vi "менеджер отчетов.vi"(8 "String":string, 10 "data":string, 11 "path":path) -> ()   [LabVIEW 2016]
uses:
  <vilib>/Utility/file.llb/Read From Spreadsheet File (string).vi
  Granule-2000AT/PC/llb/Library.lvlib
panel:
  out "Waveform Graph":dbl[](graph)
  in  "диски":string(combo)
  out "PA1":string[](array[string])
  out "TP_gas":string[](array[string])
  out "TP roller":string[](array[string])
  out "TP 2.2":string[](array[string])
  out "TP 2.1":string[](array[string])
  out "TP 1.2":string[](array[string])
  out "TP_1.1":string[](array[string])
  out "PT3":string[](array[string])
  out "PT2":string[](array[string])
  out "PT1":string[](array[string])
  out "PE3":string[](array[string])
  out "PE2":string[](array[string])
  out "PE 1":string[](array[string])
  out "SP_speed_заг":string[](array[string])
  out "SP_speed_плазматрон":string[](array[string])
  out "V_заг":string[](array[string])
  out "U_ist":string[](array[string])
  out "I_ist":string[](array[string])
  out "PV":string[](array[string])
  out "data":string[](array[string])
  out "errors":string[][](array[string])
  out "all rows":string[][](array[string])
  in  "Изделия":string(combo)
  in  "Tab Control":T1(tab)
  out "PV зазор":cluster{"data dbl":dbl[], dbl[]}(graph)
  out "Speed":cluster{"data dbl":dbl[], dbl[]}[](graph)
  out "Rotation":cluster{"data dbl":dbl[], dbl[]}(graph)
  out "I_ист":cluster{"data dbl":dbl[], dbl[]}(graph)
  out "U_ист":cluster{"data dbl":dbl[], dbl[]}(graph)
  out "Vakuum":cluster{"data dbl":dbl[], dbl[]}[](graph)
  out "Temperature":cluster{"data dbl":dbl[], dbl[]}[](graph)
  out "Presure":cluster{"data dbl":dbl[], dbl[]}[](graph)
  out "Status":u8(slide) scale=0.0..4.0
  in  "Open Button":bool
  in  "Process Stop Button":bool
  in  "Blank Button":bool
  in  "Copy Button":bool
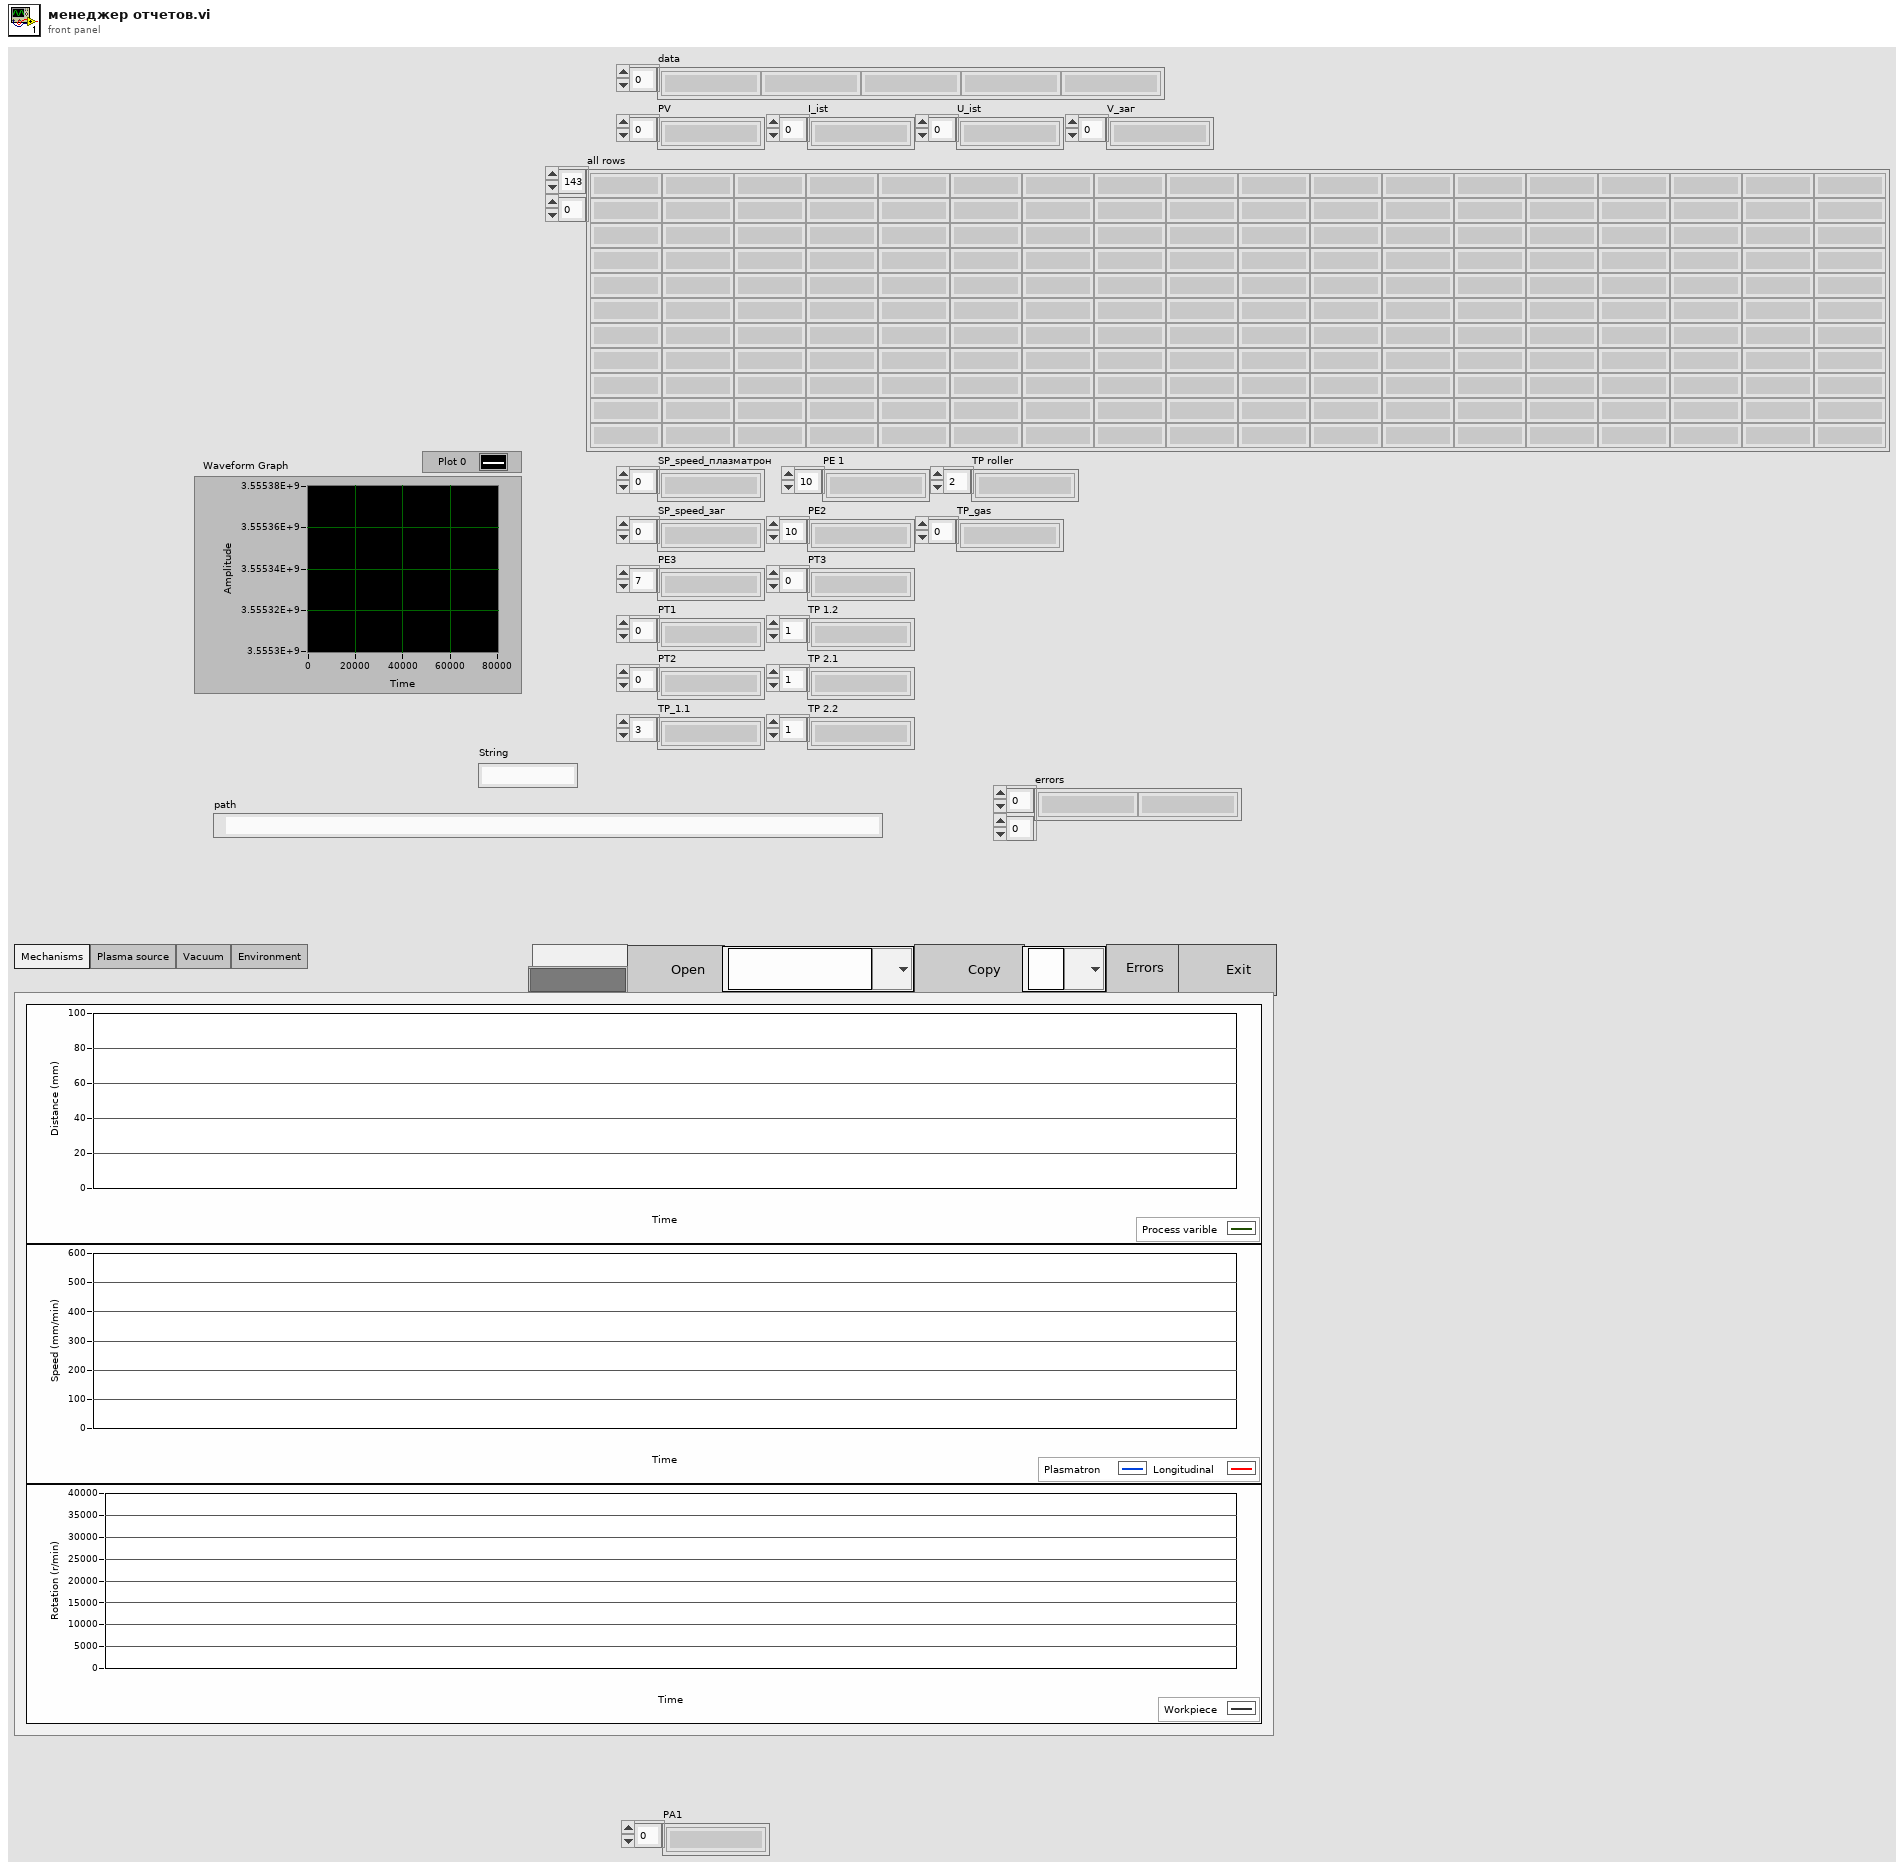
[diagram p1: front panel]
types:
  T1 = enum32{"Mechanisms", "Plasma source", "Vacuum", "Environment"}
  T2 = cluster{"String":string, "String":string, "String":string, cluster{"data dbl":dbl[], dbl[]}, cluster{"data dbl":dbl[], dbl[]}[], cluster{"data dbl":dbl[], dbl[]}}
  T3 = cluster{"String":string, "String":string, "String":string, cluster{"data dbl":dbl[], dbl[]}[], cluster{"data dbl":dbl[], dbl[]}[]}
  T4 = cluster{"String":string, "String":string, cluster{"data dbl":dbl[], dbl[]}, cluster{"data dbl":dbl[], dbl[]}, "String":string}
  T5 = cluster{"String":string, "String":string, "String":string, cluster{"data dbl":dbl[], dbl[]}[]}
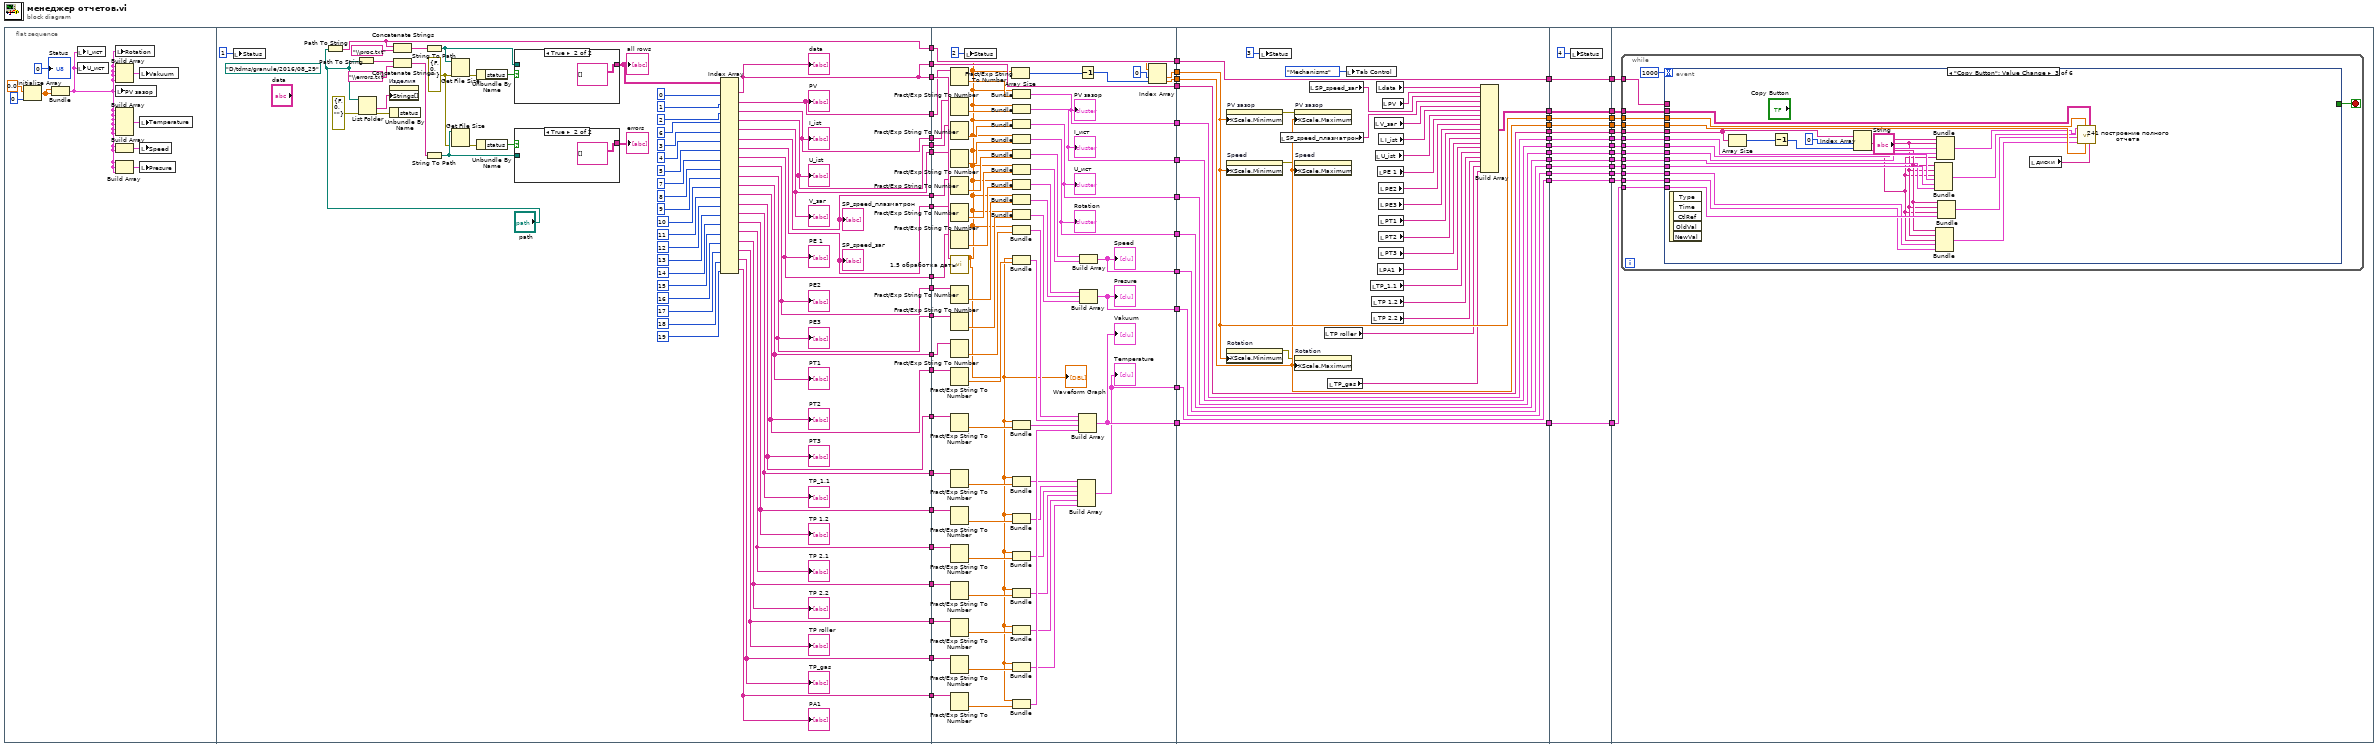
[diagram p0: block diagram]
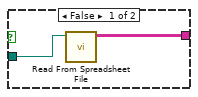
[diagram p2: hidden frame]
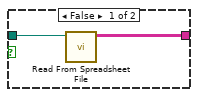
[diagram p3: hidden frame]
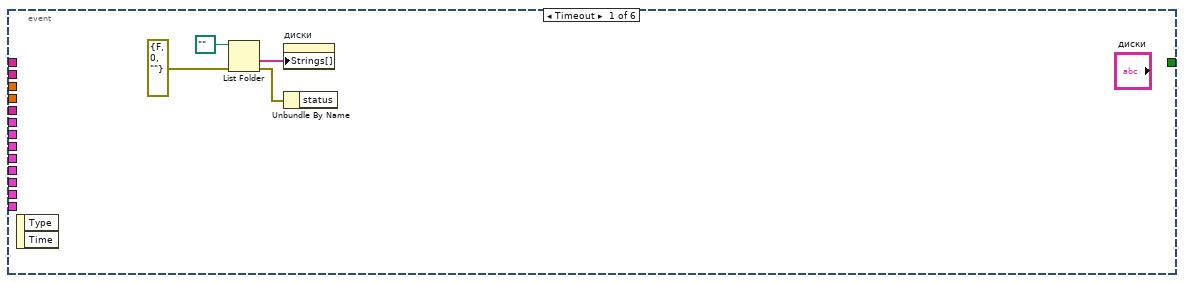
[diagram p4: hidden frame]
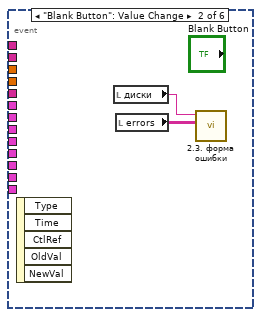
[diagram p5: hidden frame]
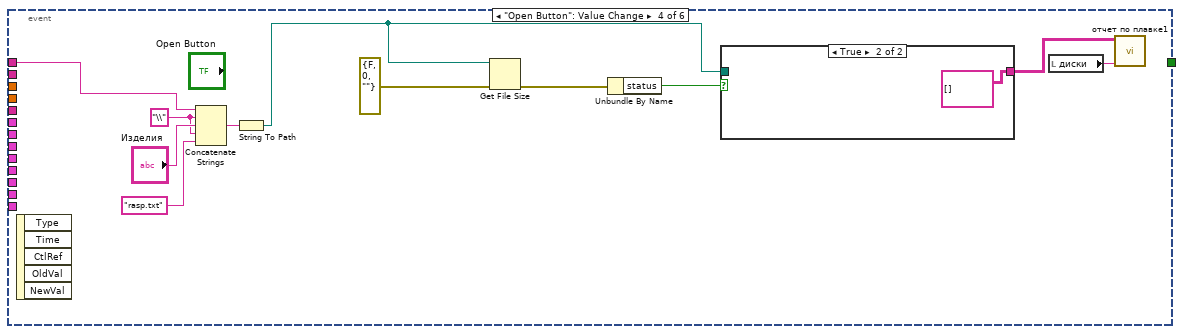
[diagram p6: hidden frame]
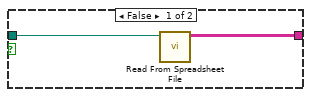
[diagram p7: hidden frame]
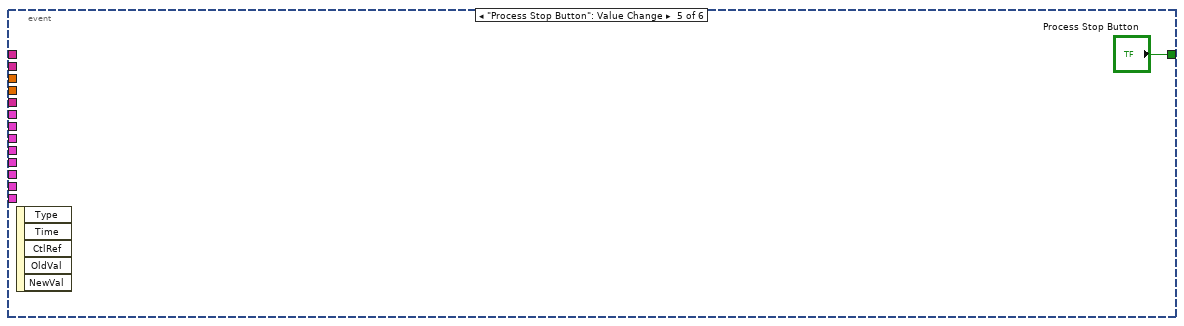
[diagram p8: hidden frame]
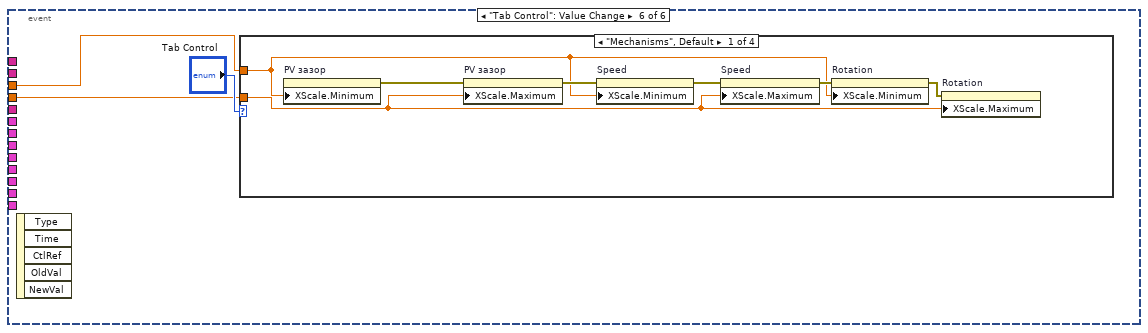
[diagram p9: hidden frame]
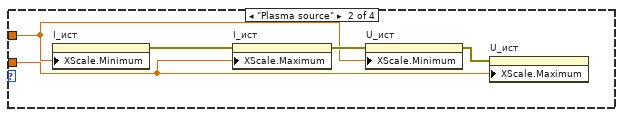
[diagram p10: hidden frame]
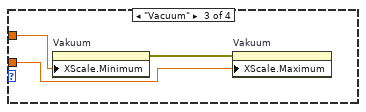
[diagram p11: hidden frame]
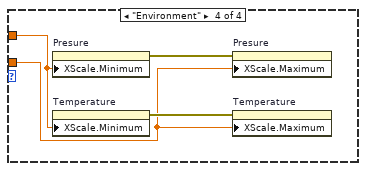
[diagram p12: hidden frame]
diagram:
  n1 = flat-sequence {
    tunnel: [w71] -> w60
    tunnel: [w93] -> w59
    tunnel: [w92] -> w58
    tunnel: [w91] -> w57
    tunnel: [w90] -> w56
    tunnel: [w89] -> w55
    tunnel: [w88] -> w54
    tunnel: [w87] -> w53
    tunnel: [w86] -> w52
    tunnel: [w85] -> w51
    tunnel: [w83] -> w50
    tunnel: [w82] -> w49
    tunnel: [w81] -> w48
    tunnel: [w80] -> w47
    tunnel: [w79] -> w46
    tunnel: [w78] -> w45
    tunnel: [w77] -> w44
    tunnel: [w76] -> w43
    tunnel: [w75] -> w42
    tunnel: [w74] -> w41
    tunnel: [w72] -> w37
    tunnel: [w71] -> w35
    tunnel: w60 -> [w206]
    tunnel: w59 -> [w205]
    tunnel: w58 -> [w200]
    tunnel: w57 -> [w198]
    tunnel: w56 -> [w194]
    tunnel: w55 -> [w192]
    tunnel: w54 -> [w189]
    tunnel: w53 -> [w188]
    tunnel: w52 -> [w186]
    tunnel: w51 -> [w184]
    tunnel: w50 -> [w175]
    tunnel: w49 -> [w174]
    tunnel: w48 -> [w173]
    tunnel: w47 -> [w172]
    tunnel: w46 -> [w155]
    tunnel: w45 -> [w154]
    tunnel: w44 -> [w153]
    tunnel: w43 -> [w152]
    tunnel: w42 -> [w151]
    tunnel: w41 -> [w150]
    tunnel: [w149] -> w40
    tunnel: [w148] -> w39
    tunnel: [w146] -> w38
    tunnel: w37 -> [w146]
    tunnel: [w145] -> w36
    tunnel: w35 -> [w145]
    tunnel: [w144] -> w22
    tunnel: [w143] -> w19
    tunnel: [w142] -> w16
    tunnel: [w141] -> w13
    tunnel: [w140] -> w10
    tunnel: [w139] -> w7
    tunnel: [w138] -> w4
    tunnel: [w137] -> w1
    tunnel: w40 -> [w242]
    tunnel: [w242] -> w34
    tunnel: w39 -> [w241]
    tunnel: [w241] -> w32
    tunnel: [w236] -> w30
    tunnel: w38 -> [w236]
    tunnel: [w216] -> w28
    tunnel: [w215] -> w26
    tunnel: w36 -> [w215]
    tunnel: [w214] -> w23
    tunnel: w22 -> [w214]
    tunnel: [w213] -> w20
    tunnel: w19 -> [w213]
    tunnel: [w212] -> w17
    tunnel: w16 -> [w212]
    tunnel: [w211] -> w14
    tunnel: w13 -> [w211]
    tunnel: [w210] -> w11
    tunnel: w10 -> [w210]
    tunnel: [w209] -> w8
    tunnel: w7 -> [w209]
    tunnel: [w208] -> w5
    tunnel: w4 -> [w208]
    tunnel: [w207] -> w2
    tunnel: w1 -> [w207]
    tunnel: w34 -> [w257]
    tunnel: [w257] -> w33
    tunnel: w32 -> [w256]
    tunnel: [w256] -> w31
    tunnel: w30 -> [w255]
    tunnel: [w255] -> w29
    tunnel: w28 -> [w254]
    tunnel: [w254] -> w27
    tunnel: w26 -> [w253]
    tunnel: [w253] -> w25
    tunnel: [w251] -> w24
    tunnel: w23 -> [w251]
    tunnel: [w250] -> w21
    tunnel: w20 -> [w250]
    tunnel: [w249] -> w18
    tunnel: w17 -> [w249]
    tunnel: [w248] -> w15
    tunnel: w14 -> [w248]
    tunnel: [w247] -> w12
    tunnel: w11 -> [w247]
    tunnel: [w246] -> w9
    tunnel: w8 -> [w246]
    tunnel: [w245] -> w6
    tunnel: w5 -> [w245]
    tunnel: [w244] -> w3
    tunnel: w2 -> [w244]
    tunnel: w33 -> [w270]
    tunnel: w31 -> [w269]
    tunnel: w29 -> [w268]
    tunnel: w27 -> [w267]
    tunnel: w25 -> [w266]
    tunnel: w24 -> [w265]
    tunnel: w21 -> [w264]
    tunnel: w18 -> [w263]
    tunnel: w15 -> [w262]
    tunnel: w12 -> [w261]
    tunnel: w9 -> [w260]
    tunnel: w6 -> [w259]
    tunnel: w3 -> [w258]
    frame #0 {
      n2 = Initialize Array(0.0, 0 ("dimension size")) -> (w67:dbl[])
      n3 = Bundle(w67, w67) -> (w63:cluster{dbl[], dbl[]})  [unwired: 1 in]
      n4 = local write "I_ист"(w63) -> ()
      n5 = local write "U_ист"(w63) -> ()
      n6 = local write "Rotation"(w63) -> ()
      n7 = Build Array(w63, w63, w63, w63) -> (w64:cluster{dbl[], dbl[]}[])
      n8 = local write "PV зазор"(w63) -> ()
      n9 = Build Array(w63, w63, w63, w63, w63, w63) -> (w62:cluster{dbl[], dbl[]}[])
      n10 = Build Array(w63, w63) -> (w66:cluster{dbl[], dbl[]}[])
      n11 = Build Array(w63, w63, w63) -> (w65:cluster{dbl[], dbl[]}[])
      n12 = local write "Vakuum"(w64) -> ()
      n13 = local write "Temperature"(w62) -> ()
      n14 = local write "Speed"(w66) -> ()
      n15 = local write "Presure"(w65) -> ()
      "Status" <- u8 0 ("Status")
    }
    frame #1 {
      w114 = errorcluster {"status"=FALSE, "code"=0, "source"=""} ("error in")
      (unwired) path "D:/tdms/granule/2016/08_29" ("path")
      n16 = local write "Status"(u8 1 ("Status")) -> ()
      n17 = Path To String(path="path") -> (string=w72:string)
      n18 = Path To String(path="path") -> (string=w125:string)
      n19 = List Folder(path="path", error in=errorcluster {"status"=FALSE, "code"=0, "source"=""}) -> (folder names=w127:string[], error out=w128:errorcluster)  [unwired: 2 in, 2 out]
      n20 = property on="Изделия" class="CmbBox"("Strings[]"=w127) -> ()  [unwired: 2 in, 2 out]
      n21 = Unbundle By Name(w128) -> ()  [unwired: 1 out]
      n22 = Concatenate Strings(w72, "\\proc.txt" ("string")) -> (w123:string)
      n23 = Concatenate Strings(w125, "\\errors.txt" ("string")) -> (w122:string)
      n24 = String To Path(string=w123) -> (path=w121:path)
      n25 = String To Path(string=w122) -> (path=w115:path)
      n26 = Get File Size(file=w121, error in=w114) -> (0:w120:errorcluster)  [unwired: 2 out]
      n27 = Get File Size(file=w115, error in=w114) -> (0:w117:errorcluster)  [unwired: 2 out]
      n28 = Unbundle By Name(w120) -> ("status"=w119:bool)
      n29 = Unbundle By Name(w117) -> ("status"=w116:bool)
      n30 = case shown="True" w119 {
        tunnel: w121 -> [w134 _]
        tunnel: [w133 string[][] [] ("all rows")] -> w113
        frame False {
          n31 = call-poly <vilib>:"Read From Spreadsheet File.vi"("file path (dialog if empty)"=w134) -> ("all rows"=w133:string[][])  [unwired: 6 in, 4 out]
        }
        frame True {
        }
      }
      "all rows" <- w113
      n32 = case shown="True" w116 {
        tunnel: w115 -> [w131 _]
        tunnel: [w130 string[][] [] ("all rows")] -> w118
        frame False {
          n33 = call-poly <vilib>:"Read From Spreadsheet File.vi"("file path (dialog if empty)"=w131) -> ("all rows"=w130:string[][])  [unwired: 6 in, 4 out]
        }
        frame True {
        }
      }
      "errors" <- w118
      n34 = Index Array(array=w113, index (col) #1=0 ("disabled index (col)"), index (col) #2=1 ("index (col)"), index (col) #3=2 ("index (col)"), index (col) #4=6 ("index (col)"), index (col) #5=3 ("index (col)"), index (col) #6=4 ("index (col)"), index (col) #7=5 ("index (col)"), index (col) #8=7 ("index (col)"), index (col) #9=8 ("index (col)"), index (col) #10=9 ("index (col)"), index (col) #11=10 ("index (col)"), index (col) #12=11 ("index (col)"), index (col) #13=12 ("index (col)"), index (col) #14=13 ("index (col)"), index (col) #15=14 ("index (col)"), index (col) #16=15 ("index (col)"), index (col) #17=16 ("index (col)"), index (col) #18=17 ("index (col)"), index (col) #19=18 ("index (col)"), index (col) #20=19 ("index (col)")) -> (element #1=w71:string[], element #2=w93:string[], element #3=w89:string[], element #4=w88:string[], element #5=w90:string[], element #6=w92:string[], element #7=w91:string[], element #8=w87:string[], element #9=w86:string[], element #10=w85:string[], element #11=w80:string[], element #12=w81:string[], element #13=w82:string[], element #14=w79:string[], element #15=w78:string[], element #16=w77:string[], element #17=w76:string[], element #18=w75:string[], element #19=w74:string[], element #20=w83:string[])  [unwired: 20 in]
      "data" <- w71
      "PV" <- w93
      "I_ist" <- w89
      "U_ist" <- w88
      "V_заг" <- w90
      "SP_speed_плазматрон" <- w92
      "SP_speed_заг" <- w91
      "PE 1" <- w87
      "PE2" <- w86
      "PE3" <- w85
      "PT1" <- w80
      "PT2" <- w81
      "PT3" <- w82
      "TP_1.1" <- w79
      "TP 1.2" <- w78
      "TP 2.1" <- w77
      "TP 2.2" <- w76
      "TP roller" <- w75
      "TP_gas" <- w74
      "PA1" <- w83
    }
    frame #2 {
      n35 = Fract/Exp String To Number(string=w205) -> (number=w201:dbl[])  [unwired: 3 in, 1 out]
      n36 = Fract/Exp String To Number(string=w192) -> (number=w191:dbl[])  [unwired: 3 in, 1 out]
      n37 = Fract/Exp String To Number(string=w189) -> (number=w190:dbl[])  [unwired: 3 in, 1 out]
      n38 = Fract/Exp String To Number(string=w194) -> (number=w193:dbl[])  [unwired: 3 in, 1 out]
      n39 = Fract/Exp String To Number(string=w200) -> (number=w199:dbl[])  [unwired: 3 in, 1 out]
      n40 = Fract/Exp String To Number(string=w198) -> (number=w197:dbl[])  [unwired: 3 in, 1 out]
      n41 = Fract/Exp String To Number(string=w188) -> (number=w187:dbl[])  [unwired: 3 in, 1 out]
      n42 = call "1.5 обработка даты.vi"("data"=w206) -> ("data dbl"=w136:dbl[])  [unwired: 10 in]
      "Waveform Graph" <- w136
      n43 = Fract/Exp String To Number(string=w186) -> (number=w185:dbl[])  [unwired: 3 in, 1 out]
      n44 = Fract/Exp String To Number(string=w184) -> (number=w183:dbl[])  [unwired: 3 in, 1 out]
      n45 = Fract/Exp String To Number(string=w172) -> (number=w168:dbl[])  [unwired: 3 in, 1 out]
      n46 = Fract/Exp String To Number(string=w173) -> (number=w169:dbl[])  [unwired: 3 in, 1 out]
      n47 = Fract/Exp String To Number(string=w174) -> (number=w170:dbl[])  [unwired: 3 in, 1 out]
      n48 = Fract/Exp String To Number(string=w155) -> (number=w161:dbl[])  [unwired: 3 in, 1 out]
      n49 = Fract/Exp String To Number(string=w154) -> (number=w160:dbl[])  [unwired: 3 in, 1 out]
      n50 = Fract/Exp String To Number(string=w153) -> (number=w159:dbl[])  [unwired: 3 in, 1 out]
      n51 = Fract/Exp String To Number(string=w152) -> (number=w158:dbl[])  [unwired: 3 in, 1 out]
      n52 = Fract/Exp String To Number(string=w151) -> (number=w156:dbl[])  [unwired: 3 in, 1 out]
      n53 = Fract/Exp String To Number(string=w150) -> (number=w157:dbl[])  [unwired: 3 in, 1 out]
      n54 = Fract/Exp String To Number(string=w175) -> (number=w171:dbl[])  [unwired: 3 in, 1 out]
      n55 = local write "Status"(u8 2 ("Status")) -> ()
      n56 = Array Size(array=w136) -> (size(s)=w203:i32)
      n57 = Bundle("data dbl"=w136, w201) -> (w144:cluster{"data dbl":dbl[], dbl[]})  [unwired: 1 in]
      "PV зазор" <- w144
      n58 = Bundle("data dbl"=w136, w191) -> (w141:cluster{"data dbl":dbl[], dbl[]})  [unwired: 1 in]
      "I_ист" <- w141
      n59 = Bundle("data dbl"=w136, w190) -> (w140:cluster{"data dbl":dbl[], dbl[]})  [unwired: 1 in]
      "U_ист" <- w140
      n60 = Bundle("data dbl"=w136, w193) -> (w142:cluster{"data dbl":dbl[], dbl[]})  [unwired: 1 in]
      "Rotation" <- w142
      n61 = Bundle("data dbl"=w136, w199) -> (w196:cluster{"data dbl":dbl[], dbl[]})  [unwired: 1 in]
      n62 = Bundle("data dbl"=w136, w197) -> (w195:cluster{"data dbl":dbl[], dbl[]})  [unwired: 1 in]
      n63 = Bundle("data dbl"=w136, w187) -> (w182:cluster{"data dbl":dbl[], dbl[]})  [unwired: 1 in]
      n64 = Bundle("data dbl"=w136, w185) -> (w181:cluster{"data dbl":dbl[], dbl[]})  [unwired: 1 in]
      n65 = Bundle("data dbl"=w136, w183) -> (w180:cluster{"data dbl":dbl[], dbl[]})  [unwired: 1 in]
      n66 = Bundle("data dbl"=w136, w168) -> (w179:cluster{"data dbl":dbl[], dbl[]})  [unwired: 1 in]
      n67 = Bundle("data dbl"=w136, w169) -> (w178:cluster{"data dbl":dbl[], dbl[]})  [unwired: 1 in]
      n68 = Bundle("data dbl"=w136, w170) -> (w177:cluster{"data dbl":dbl[], dbl[]})  [unwired: 1 in]
      n69 = Bundle("data dbl"=w136, w161) -> (w167:cluster{"data dbl":dbl[], dbl[]})  [unwired: 1 in]
      n70 = Bundle("data dbl"=w136, w160) -> (w166:cluster{"data dbl":dbl[], dbl[]})  [unwired: 1 in]
      n71 = Bundle("data dbl"=w136, w159) -> (w165:cluster{"data dbl":dbl[], dbl[]})  [unwired: 1 in]
      n72 = Bundle("data dbl"=w136, w158) -> (w164:cluster{"data dbl":dbl[], dbl[]})  [unwired: 1 in]
      n73 = Bundle("data dbl"=w136, w156) -> (w163:cluster{"data dbl":dbl[], dbl[]})  [unwired: 1 in]
      n74 = Bundle("data dbl"=w136, w157) -> (w162:cluster{"data dbl":dbl[], dbl[]})  [unwired: 1 in]
      n75 = Bundle("data dbl"=w136, w171) -> (w176:cluster{"data dbl":dbl[], dbl[]})  [unwired: 1 in]
      n76 = Build Array(w167, w166, w165, w164, w163, w162) -> (w137:cluster{"data dbl":dbl[], dbl[]}[])
      "Temperature" <- w137
      n77 = Decrement(x=w203) -> (x-1=w202:i32)
      n78 = Build Array(w179, w178, w177, w176) -> (w139:cluster{"data dbl":dbl[], dbl[]}[])
      "Vakuum" <- w139
      n79 = Build Array(w182, w181, w180) -> (w138:cluster{"data dbl":dbl[], dbl[]}[])
      "Presure" <- w138
      n80 = Build Array(w196, w195) -> (w143:cluster{"data dbl":dbl[], dbl[]}[])
      "Speed" <- w143
      n81 = Index Array(array=w136, index #1=0 ("index"), index #2=w202) -> (element #1=w149:dbl, element #2=w148:dbl)
    }
    frame #3 {
      n82 = property on="PV зазор" class="XYGraph (strict)"("XScale.Minimum"=w242) -> (error out=w240:errorcluster)  [unwired: 2 in, 1 out]
      n83 = property on="Speed" class="XYGraph (strict)"("XScale.Minimum"=w242) -> (error out=w239:errorcluster)  [unwired: 2 in, 1 out]
      n84 = property on="Rotation" class="XYGraph (strict)"("XScale.Minimum"=w242) -> (error out=w238:errorcluster)  [unwired: 2 in, 1 out]
      n85 = local write "Status"(u8 3 ("Status")) -> ()
      n86 = local read "SP_speed_плазматрон"() -> (w232:string[])
      n87 = property on="PV зазор" class="XYGraph (strict)"(error in=w240, "XScale.Maximum"=w241) -> ()  [unwired: 1 in, 2 out]
      n88 = property on="Speed" class="XYGraph (strict)"(error in=w239, "XScale.Maximum"=w241) -> ()  [unwired: 1 in, 2 out]
      n89 = property on="Rotation" class="XYGraph (strict)"(error in=w238, "XScale.Maximum"=w241) -> ()  [unwired: 1 in, 2 out]
      n90 = local read "SP_speed_заг"() -> (w233:string[])
      n91 = local read "TP roller"() -> (w218:string[])
      n92 = local read "TP_gas"() -> (w217:string[])
      n93 = local write "Tab Control"(T1."Mechanisms" ("Tab Control")) -> ()
      n94 = local read "TP_1.1"() -> (w221:string[])
      n95 = local read "TP 1.2"() -> (w220:string[])
      n96 = local read "TP 2.2"() -> (w219:string[])
      n97 = local read "V_заг"() -> (w231:string[])
      n98 = local read "U_ist"() -> (w229:string[])
      n99 = local read "data"() -> (w235:string[])
      n100 = local read "PE 1"() -> (w228:string[])
      n101 = local read "PA1"() -> (w222:string[])
      n102 = local read "I_ist"() -> (w230:string[])
      n103 = local read "PE2"() -> (w227:string[])
      n104 = local read "PE3"() -> (w226:string[])
      n105 = local read "PT1"() -> (w225:string[])
      n106 = local read "PT2"() -> (w224:string[])
      n107 = local read "PT3"() -> (w223:string[])
      n108 = local read "PV"() -> (w234:string[])
      n109 = Build Array(w235, w234, w233, w232, w231, w230, w229, w228, w227, w226, w225, w224, w223, w222, w221, w220, w219, w218, w217) -> (w216:string[][])
    }
    frame #4 {
      n110 = local write "Status"(u8 4 ("Status")) -> ()
    }
    frame #5 {
      n111 = while {
        tunnel: w270 -> [w285]
        tunnel: w269 -> [w284]
        tunnel: w268 -> [w282]
        tunnel: w267 -> [w280]
        tunnel: w266 -> [w279]
        tunnel: w265 -> [w278]
        tunnel: w264 -> [w277]
        tunnel: w263 -> [w276]
        tunnel: w262 -> [w275]
        tunnel: w261 -> [w274]
        tunnel: w260 -> [w273]
        tunnel: w259 -> [w272]
        tunnel: w258 -> [w271]
        stop <- w281 stop-if-true
        n112 = event shown="[2] \"Copy Button\": Value Change" {
          selector: _ -> [_ _ _ _ _ _]
          dyn-events: _ -> [_ _ _ _ _ _]
          timeout: 1000 -> [_ _ _ _ _ _]
          tunnel: w285 -> [_ _ w312 _ _ w331]
          tunnel: w284 -> [_ _ w313 _ _ w330]
          tunnel: w282 -> [_ _ _ w325 _ _]
          tunnel: [_ _ _ _ "Process Stop Button" _] -> w281
          tunnel: w280 -> [_ _ w314 _ _ _]
          tunnel: w279 -> [_ _ w310 _ _ _]
          tunnel: w278 -> [_ _ w306 _ _ _]
          tunnel: w277 -> [_ _ w305 _ _ _]
          tunnel: w276 -> [_ _ w304 _ _ _]
          tunnel: w275 -> [_ _ w302 _ _ _]
          tunnel: w274 -> [_ _ w301 _ _ _]
          tunnel: w273 -> [_ _ w299 _ _ _]
          tunnel: w272 -> [_ _ w295 _ _ _]
          tunnel: w271 -> [_ _ w294 _ _ _]
          event Timeout {
            n113 = event-data() -> ()  [unwired: 1 in, 2 out]
            n114 = List Folder(path=path "", error in=errorcluster {"status"=FALSE, "code"=0, "source"=""}) -> (folder names=w288:string[], error out=w286:errorcluster)  [unwired: 2 in, 2 out]
            n115 = property on="диски" class="CmbBox"("Strings[]"=w288) -> ()  [unwired: 2 in, 2 out]
            n116 = Unbundle By Name(w286) -> ()  [unwired: 1 out]
          }
          event "Blank Button": Value Change {
            n117 = event-data() -> ()  [unwired: 1 in, 5 out]
            n118 = local read "диски"() -> (w291:string)
            n119 = local read "errors"() -> (w290:string[][])
            n120 = call "2.3. форма ошибки.vi"("errors"=w290, "disk"=w291) -> ()  [unwired: 10 in]
          }
          event "Copy Button": Value Change {
            n121 = event-data() -> ()  [unwired: 1 in, 5 out]
            n122 = Array Size(array=w310) -> (size(s)=w308:i32)
            n123 = Decrement(x=w308) -> (x-1=w307:i32)
            n124 = Index Array(array=w310, index #1=0 ("index"), index #2=w307) -> (element #1=w296:string, element #2=w297:string)
            n125 = Bundle("String"=w297, "String"=w296, "String"="String", w306, w305, w304) -> (w303:T2)  [unwired: 1 in]
            n126 = Bundle("String"=w297, "String"=w296, "String"="String", w295, w294) -> (w293:T3)  [unwired: 1 in]
            n127 = Bundle("String"=w297, "String"=w296, w302, w301, "String"="String") -> (w300:T4)  [unwired: 1 in]
            n128 = Bundle("String"=w297, "String"=w296, "String"="String", w299) -> (w298:T5)  [unwired: 1 in]
            n129 = local read "диски"() -> (w311:string)
            n130 = call "241 построение полного отчета.vi"("disk"=w311, "appended array"=w314, "X Scale.Range:Maximum"=w313, "X Scale.Range:Minimum"=w312, "Cluster 4"=w293, "Cluster 3"=w298, "Cluster 2"=w300, "Cluster"=w303) -> ()  [unwired: 4 in]
          }
          event "Open Button": Value Change {
            w323 = "\\" ("string")
            n131 = event-data() -> ()  [unwired: 1 in, 5 out]
            n132 = Concatenate Strings(w325, w323, "Изделия", w323, "rasp.txt" ("string")) -> (w321:string)
            n133 = String To Path(string=w321) -> (path=w317:path)
            n134 = Get File Size(file=w317, error in=errorcluster {"status"=FALSE, "code"=0, "source"=""}) -> (0:w319:errorcluster)  [unwired: 2 out]
            n135 = Unbundle By Name(w319) -> ("status"=w318:bool)
            n136 = case shown="True" w318 {
              tunnel: w317 -> [w327 _]
              tunnel: [w326 string[][] [] ("all rows")] -> w316
              frame False {
                n137 = call-poly <vilib>:"Read From Spreadsheet File.vi"("file path (dialog if empty)"=w327) -> ("all rows"=w326:string[][])  [unwired: 6 in, 4 out]
              }
              frame True {
              }
            }
            n138 = local read "диски"() -> (w315:string)
            n139 = call "отчет по плавке1.vi"("disk"=w315, "rasp"=w316) -> ()  [unwired: 10 in]
          }
          event "Process Stop Button": Value Change {
            n140 = event-data() -> ()  [unwired: 1 in, 5 out]
          }
          event "Tab Control": Value Change {
            n141 = event-data() -> ()  [unwired: 1 in, 5 out]
            n142 = case shown="\"Mechanisms\", Default" "Tab Control" {
              tunnel: w331 -> [w334 w341 w346 w349]
              tunnel: w330 -> [w333 w340 w345 w348]
              frame "Mechanisms", Default {
                n143 = property on="PV зазор" class="XYGraph (strict)"("XScale.Minimum"=w334) -> (error out=w338:errorcluster)  [unwired: 2 in, 1 out]
                n144 = property on="PV зазор" class="XYGraph (strict)"(error in=w338, "XScale.Maximum"=w333) -> (error out=w337:errorcluster)  [unwired: 1 in, 1 out]
                n145 = property on="Speed" class="XYGraph (strict)"(error in=w337, "XScale.Minimum"=w334) -> (error out=w339:errorcluster)  [unwired: 1 in, 1 out]
                n146 = property on="Speed" class="XYGraph (strict)"(error in=w339, "XScale.Maximum"=w333) -> (error out=w335:errorcluster)  [unwired: 1 in, 1 out]
                n147 = property on="Rotation" class="XYGraph (strict)"(error in=w335, "XScale.Minimum"=w334) -> (error out=w336:errorcluster)  [unwired: 1 in, 1 out]
                n148 = property on="Rotation" class="XYGraph (strict)"(error in=w336, "XScale.Maximum"=w333) -> ()  [unwired: 1 in, 2 out]
              }
              frame "Plasma source" {
                n149 = property on="I_ист" class="XYGraph (strict)"("XScale.Minimum"=w341) -> (error out=w344:errorcluster)  [unwired: 2 in, 1 out]
                n150 = property on="I_ист" class="XYGraph (strict)"(error in=w344, "XScale.Maximum"=w340) -> (error out=w342:errorcluster)  [unwired: 1 in, 1 out]
                n151 = property on="U_ист" class="XYGraph (strict)"(error in=w342, "XScale.Minimum"=w341) -> (error out=w343:errorcluster)  [unwired: 1 in, 1 out]
                n152 = property on="U_ист" class="XYGraph (strict)"(error in=w343, "XScale.Maximum"=w340) -> ()  [unwired: 1 in, 2 out]
              }
              frame "Vacuum" {
                n153 = property on="Vakuum" class="XYGraph (strict)"("XScale.Minimum"=w346) -> (error out=w347:errorcluster)  [unwired: 2 in, 1 out]
                n154 = property on="Vakuum" class="XYGraph (strict)"(error in=w347, "XScale.Maximum"=w345) -> ()  [unwired: 1 in, 2 out]
              }
              frame "Environment" {
                n155 = property on="Presure" class="XYGraph (strict)"("XScale.Minimum"=w349) -> (error out=w351:errorcluster)  [unwired: 2 in, 1 out]
                n156 = property on="Temperature" class="XYGraph (strict)"("XScale.Minimum"=w349) -> (error out=w350:errorcluster)  [unwired: 2 in, 1 out]
                n157 = property on="Presure" class="XYGraph (strict)"(error in=w351, "XScale.Maximum"=w348) -> ()  [unwired: 1 in, 2 out]
                n158 = property on="Temperature" class="XYGraph (strict)"(error in=w350, "XScale.Maximum"=w348) -> ()  [unwired: 1 in, 2 out]
              }
            }
          }
        }
      }
    }
  }
